vi "Save Sequence.vi"(8 "Error In":errorcluster, 10 "Selected Path":path, 11 "CS++SeqEditor in":refnum<class "CS++SeqEditor.lvclass">) -> (0 "Error Out":errorcluster, 3 "CS++SeqEditor out":refnum<class "CS++SeqEditor.lvclass">)   [LabVIEW 2016, in "CS++SeqEditor.lvlib" / "CS++SeqEditor.lvclass"]
doc: "Save sequence to file."
uses:
  CS++SeqEditor.lvclass
  CS++SeqEditor.lvclass/CS++SeqEditor.ctl
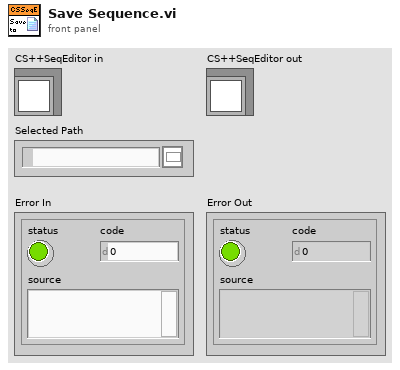
[diagram p1: front panel]
types:
  T1 = enum16{"open", "replace", "create", "open or create", "replace or create", "replace or create with confirmation"}
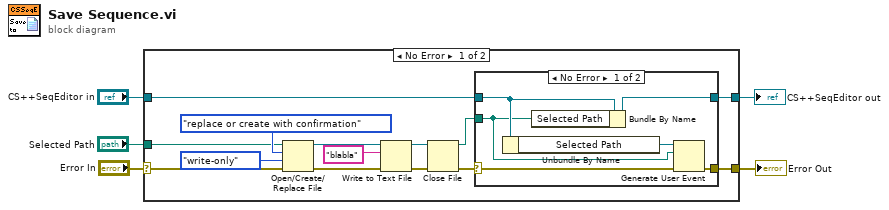
[diagram p0: block diagram]
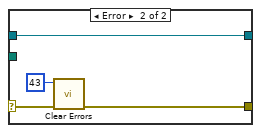
[diagram p2: hidden frame]
diagram:
  n1 = case shown="No Error" "Error In" {
    selector: "Error In" -> [w12 w31]
    tunnel: [w8 w31] -> w4
    tunnel: [w18 w30] -> w2
    tunnel: "CS++SeqEditor in" -> [w19 w30]
    tunnel: "Selected Path" -> [w7 _]
    frame No Error {
      n2 = Open/Create/Replace File(file path (use dialog)=w7, error in=w12, operation (0:open)=T1."replace or create with confirmation", access (0:read/write)=enum16{"read/write", "read-only", "write-only"}."write-only") -> (refnum out=w15:refnum<file>, error out=w14:errorcluster)  [unwired: 2 in, 1 out]
      n3 = Write to Text File(file (use dialog)=w15, text="blabla", error in=w14) -> (refnum out=w10:refnum<file>, error out=w11:errorcluster)  [unwired: 1 in, 1 out]
      n4 = Close File(refnum=w10, error in=w11) -> (path=w6:path, error out=w9:errorcluster)
      n5 = case shown="No Error" w9 {
        selector: w9 -> [w21 w28]
        tunnel: w19 -> [w24 w29]
        tunnel: [w25 w29] -> w18
        tunnel: w6 -> [w22 _]
        tunnel: [w20 w27] -> w8
        frame No Error {
          n6 = Unbundle By Name(w24) -> ("Selected Path"=w23:refnum<user-event>)
          n7 = Bundle By Name(cluster=w24, "Selected Path"=w22) -> (w25:refnum<class "CS++SeqEditor.lvclass">)
          n8 = Generate User Event(user event=w23, event data cluster=w22, error in=w21) -> (error out=w20:errorcluster)  [unwired: 1 in, 1 out]
        }
        frame Error {
          n9 = call <vilib>:"Clear Errors.vi"("error in (no error)"=w28, "specific error code to clear (0: all)"=43) -> ("error out"=w27:errorcluster)  [unwired: 4 in, 1 out]
        }
      }
    }
    frame Error {
    }
  }
  "Error Out" <- w4
  "CS++SeqEditor out" <- w2
